vi "gen_s_v0.vi"() -> ()   [LabVIEW 2009]
uses:
  <vilib>/Platform/portaccess.llb/Out Port8.vi
  <vilib>/Platform/portaccess.llb/In Port8.vi
panel:
  out "Waveform Graph":u32[](graph)
  out "Numeric":dbl
  in  "stop":bool
  out "Waveform Chart":u32(graph)
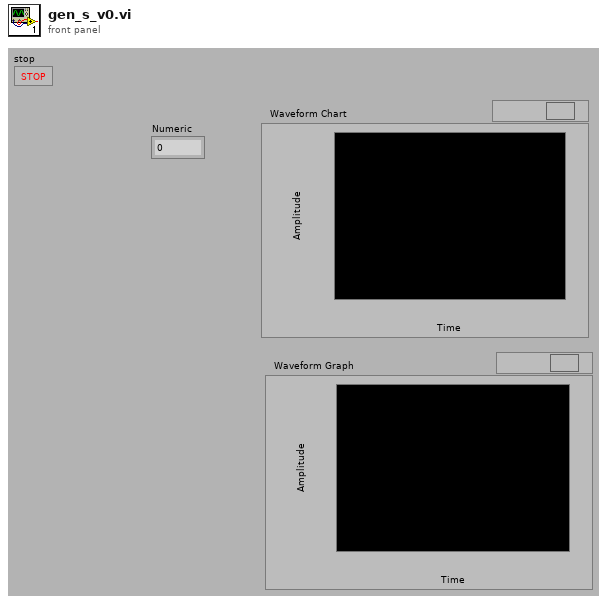
[diagram p1: front panel]
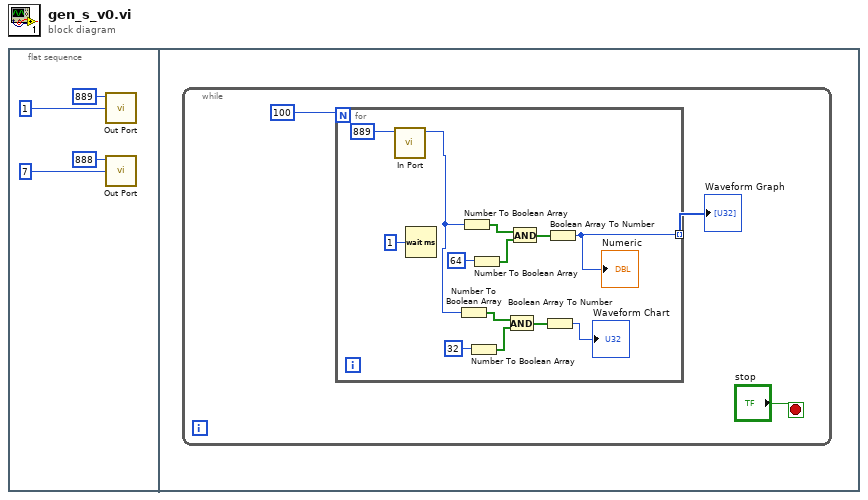
[diagram p0: block diagram]
diagram:
  n1 = flat-sequence {
    frame #0 {
      n2 = call-poly <vilib>:"Out Port.vi"("write value"=u8 1, "address"=i16 889) -> ()  [unwired: 7 in, 1 out]
      n3 = call-poly <vilib>:"Out Port.vi"("write value"=u8 7, "address"=i16 888) -> ()  [unwired: 7 in, 1 out]
    }
    frame #1 {
      n4 = while {
        stop <- "stop" stop-if-true
        n5 = for {
          N: 100 -> [_]
          tunnel: [w14] -> w5 mode=indexing
          n6 = call-poly <vilib>:"In Port.vi"("address"=i16 889) -> ("data read"=w8:i8)  [unwired: 7 in, 1 out]
          n7 = Wait (ms)(milliseconds to wait=u32 1) -> ()  [unwired: 1 out]
          n8 = Number To Boolean Array(number=w8) -> (Boolean array=w13:bool[])
          n9 = Number To Boolean Array(number=w8) -> (Boolean array=w18:bool[])
          n10 = Number To Boolean Array(number=u32 32 ("milliseconds to wait")) -> (Boolean array=w11:bool[])
          n11 = Number To Boolean Array(number=u32 64 ("milliseconds to wait")) -> (Boolean array=w16:bool[])
          n12 = And(x=w13, y=w11) -> (x .and. y?=w10:bool[])
          n13 = And(x=w18, y=w16) -> (x .and. y?=w15:bool[])
          n14 = Boolean Array To Number(Boolean array=w10) -> (number=→"Waveform Chart":u32)
          n15 = Boolean Array To Number(Boolean array=w15) -> (number=w14:u32)
          "Numeric" <- w14
        }
        "Waveform Graph" <- w5
      }
    }
  }
